vi "Initialize Event References.vi"(8 "error in (no error)":errorcluster) -> (0 "error out":errorcluster, 3 "Event-References":T1)   [LabVIEW 2018, in "Copy of Actor.lvclass"]
uses:
  Copy of Actor.lvclass
  Event-References.ctl
  Stop.ctl
  Launched.ctl
  Some Request.ctl
  Some Response.ctl
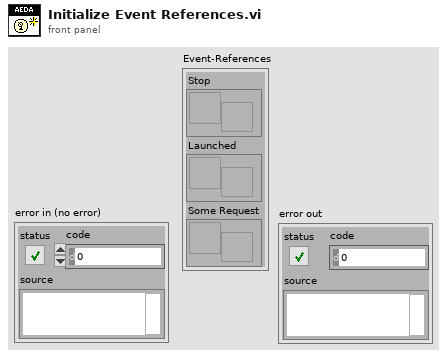
[diagram p1: front panel]
types:
  T1 = typedef "Copy of Actor.lvclass/Event-References.ctl" = cluster{"Stop":refnum<user-event>, "Launched":refnum<user-event>, "Some Request":refnum<user-event>}
  T2 = typedef "Copy of Actor.lvclass/Some Request.ctl" = string
  T3 = cluster{"Some Request":T2, "Some Response":refnum<user-event>}
  T4 = typedef "Copy of Actor.lvclass/Launched.ctl" = cluster{"Launched State":refnum<class "Copy of Actor.lvclass">}
  T5 = typedef "Copy of Actor.lvclass/Stop.ctl" = enum16{"Normal", "Emergency"}
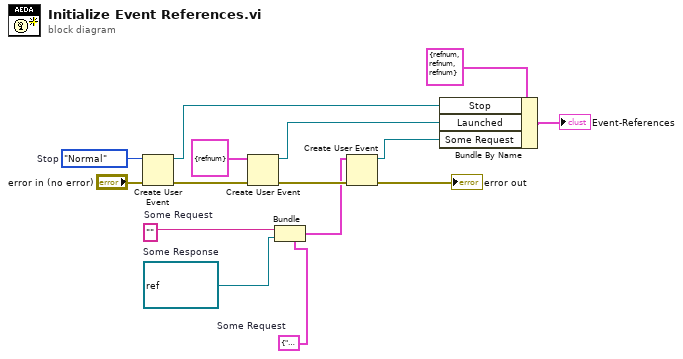
[diagram p0: block diagram]
diagram:
  w1 = T3 {"Some Request"="", "Some Response"=refnum}  # Some Request
  w4 = refnum<user-event> refnum  # Some Response
  w5 = T2 ""  # Some Request
  w13 = Stop."Normal"  # Stop
  n1 = Create User Event(user event datatype=w13, error in="error in (no error)") -> (user event=w10:refnum<user-event>, error out=w15:errorcluster)
  n2 = Create User Event(user event datatype=T4 {"Launched State"=refnum} ("Launched"), error in=w15) -> (user event=w9:refnum<user-event>, error out=w7:errorcluster)
  n3 = Bundle(cluster=w1, "Some Request"=w5, "Some Response"=w4) -> (w3:T3)
  n4 = Create User Event(user event datatype=w3, error in=w7) -> (user event=w2:refnum<user-event>, error out=→"error out":errorcluster)
  n5 = Bundle By Name(cluster=T1 {"Stop"=refnum, "Launched"=refnum, "Some Request"=refnum} ("Actor-Events"), "Stop"=w10, "Launched"=w9, "Some Request"=w2) -> (→"Event-References":T1)
